vi "Write Numeric.vi"(8 "error in (no error)":errorcluster, 10 "Numeric":dbl, 11 "myClassWOPropFolder in":refnum<class "myClassWOPropFolder.lvclass">) -> (0 "error out":errorcluster, 3 "myClassWOPropFolder out":refnum<class "myClassWOPropFolder.lvclass">)   [LabVIEW 2017, in "myClassWOPropFolder.lvclass"]
uses:
  myClassWOPropFolder.lvclass
  myClassWOPropFolder.lvclass/myClassWOPropFolder.ctl
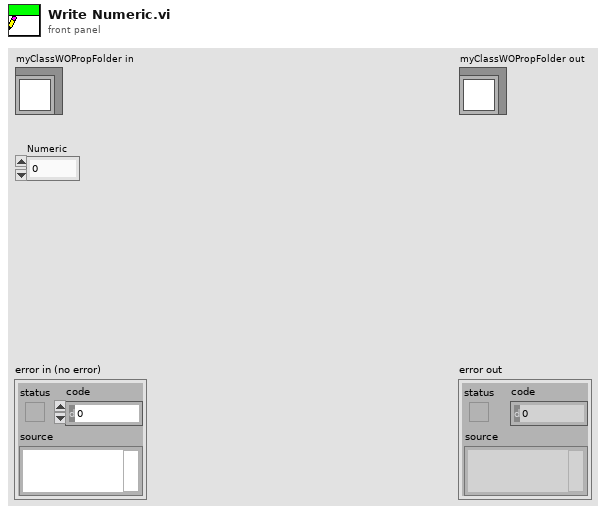
[diagram p1: front panel]
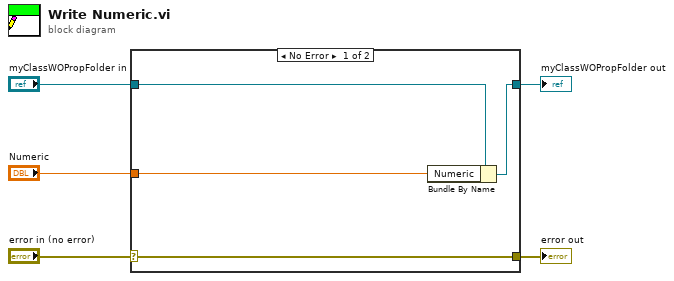
[diagram p0: block diagram]
diagram:
  n1 = case shown="No Error" "error in (no error)" {
    selector: "error in (no error)" -> [w9 w10]
    tunnel: [w9 w10] -> w4
    tunnel: [w7 w11] -> w2
    tunnel: "myClassWOPropFolder in" -> [w8 w11]
    tunnel: "Numeric" -> [w6 _]
    frame No Error {
      n2 = Bundle By Name(cluster=w8, "Numeric"=w6) -> (w7:refnum<class "myClassWOPropFolder.lvclass">)
    }
    frame Error {
    }
  }
  "error out" <- w4
  "myClassWOPropFolder out" <- w2
